vi "Fill From.vi"(5 "Col":i32, 6 "Attributes":T1, 7 "Row":i32, 8 "error in (no error)":errorcluster, 10 "Char":string, 11 "TermBuffer in":refnum<class "TermBuffer.lvclass">) -> (0 "error out":errorcluster, 3 "TermBuffer out":refnum<class "TermBuffer.lvclass">)   [LabVIEW 2020, in "Terminal.lvlib" / "TermBuffer.lvclass"]
uses:
  TermBuffer.lvclass
  TermBuffer.lvclass/TermBuffer.ctl
  TermLine/TermLine.lvclass
  Text Attributes.ctl
  Terminal.lvlib
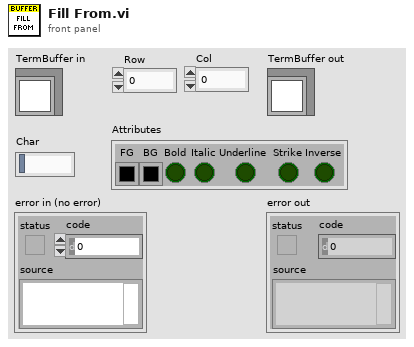
[diagram p1: front panel]
types:
  T1 = typedef "Terminal.lvlib/Text Attributes.ctl" = cluster{"FG":u32, "BG":u32, "Bold":bool, "Italic":bool, "Underline":bool, "Strike":bool, "Inverse":bool}
  T2 = typedef "Terminal.lvlib/TermBuffer.lvclass/Ref Data.ctl" = cluster{"Lines":refnum<class "TermLine.lvclass">[], "Rows":i32, "Cols":i32}
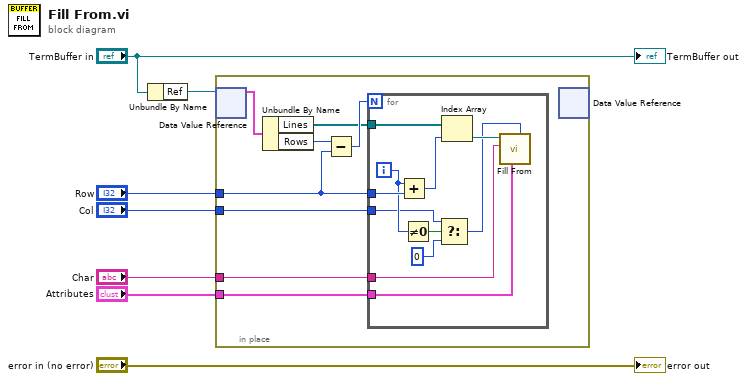
[diagram p0: block diagram]
diagram:
  n1 = Unbundle By Name("TermBuffer in") -> ("Ref"=w6:refnum<data-value>)
  n2 = in-place {
    in-place-border: "Row" -> [w11]
    in-place-border: "Col" -> [w10]
    in-place-border: "Char" -> [w9]
    in-place-border: "Attributes" -> [w8]
    n3 = in-place-dvr #1(w6) -> (w15:T2)  [unwired: 1 out]
    n4 = Unbundle By Name(w15) -> ("Lines"=w12:refnum<class "TermLine.lvclass">[], "Rows"=w14:i32)
    n5 = Subtract(x=w14, y=w11) -> (x-y=w13:i32)
    n6 = for {
      N: w13 -> [_]
      tunnel: w12 -> [w25]
      tunnel: w11 -> [w26]
      tunnel: w10 -> [w21]
      tunnel: w9 -> [w17]
      tunnel: w8 -> [w16]
      i -> [w23]
      n7 = Add(x=w23, y=w26) -> (x+y=w24:i32)
      n8 = Not Equal To 0?(x=w23) -> (x != 0?=w22:bool)
      n9 = Select(t=w21, s=w22, f=0) -> (s? t:f=w18:i32)
      n10 = Index Array(array=w25, index=w24) -> (element=w19:refnum<class "TermLine.lvclass">)
      n11 = call "Fill From.vi"("Col"=w18, "Attributes"=w16, "Char"=w17, "TermLine in"=w19) -> ()  [unwired: 6 in, 2 out]
    }
    n12 = in-place-dvr #1() -> ()  [unwired: 1 in, 2 out]
  }
  "error out" <- "error in (no error)"
  "TermBuffer out" <- "TermBuffer in"
